vi "Hide the SessionId.vi"(11 "error in (no error)":errorcluster) -> (15 "error out":errorcluster)   [LabVIEW 2021, in "G Plug-in Migrator.lvlib"]
uses:
  G Plug-in Migrator.lvlib
  Path Functions/Path Functions.lvlib
  Migrator Reusables/Migrator Reusables.lvlib
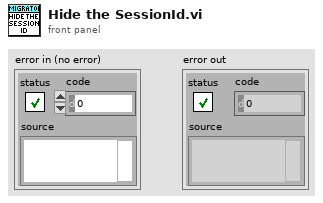
[diagram p1: front panel]
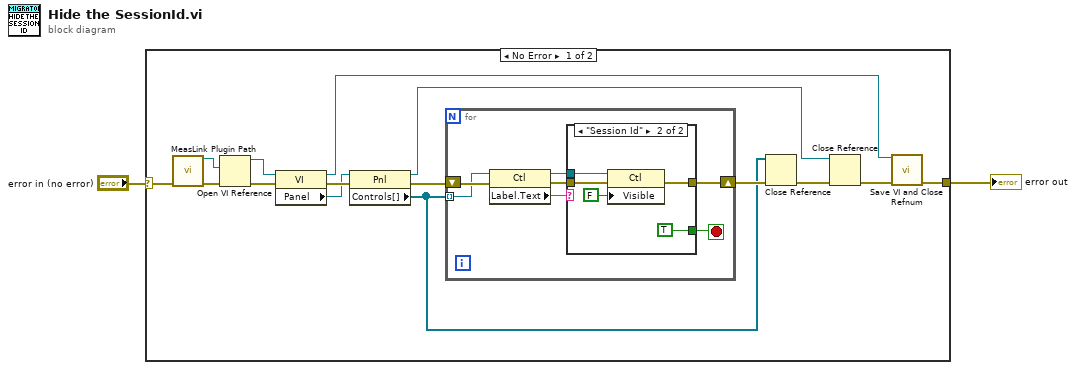
[diagram p0: block diagram]
diagram:
  n1 = case shown="No Error" "error in (no error)" {
    selector: "error in (no error)" -> [w17 w31]
    tunnel: [w4 w31] -> w2
    frame No Error {
      n2 = call "MeasLink Plugin Path.vi"("error in (no error)"=w17) -> ("New Code Module"=w16:path, "error out"=w15:errorcluster)  [unwired: 2 in, 11 out]
      n3 = Open VI Reference(vi path=w16, error in (no error)=w15) -> (vi reference=w12:refnum<vi>, error out=w14:errorcluster)  [unwired: 4 in]
      n4 = property class="VI"(reference=w12, error in=w14) -> (reference out=w3:refnum<vi>, error out=w13:errorcluster, "Panel"=w11:refnum<vi>)
      n5 = property class="Pnl"(reference=w11, error in=w13) -> (reference out=w6:refnum<vi>, error out=w10:errorcluster, "Controls[]"=w7:refnum<vi>[])
      n6 = for {
        tunnel: w7 -> [w23] mode=indexing
        shift-right: [w19] -> w9
        shift-left: w10 -> [w24]
        stop <- w18 stop-if-true
        n7 = property class="Ctl"(reference=w23, error in=w24) -> (reference out=w21:refnum<vi>, error out=w20:errorcluster, "Label.Text"=w22:string)
        n8 = case shown="\"Session Id\"" w22 {
          tunnel: w21 -> [_ w30]
          tunnel: w20 -> [w25 w29]
          tunnel: [w25 w27] -> w19
          tunnel: [_ TRUE] -> w18
          frame Default {
          }
          frame "Session Id" {
            n9 = property class="Ctl"(reference=w30, error in=w29, "Visible"=FALSE) -> (error out=w27:errorcluster)  [unwired: 1 out]
          }
        }
      }
      n10 = Close Reference(reference=w7, error in (no error)=w9) -> (error out=w8:errorcluster)
      n11 = Close Reference(reference=w6, error in (no error)=w8) -> (error out=w5:errorcluster)
      n12 = call "Save VI and Close Refnum.vi"("VI Refnum"=w3, "error in"=w5) -> ("error out"=w4:errorcluster)  [unwired: 13 in]
    }
    frame Error {
    }
  }
  "error out" <- w2
